vi "Read Stdout.vi"(8 "error in":errorcluster, 10 "byte count":i32, 11 "pipe in":T1) -> (0 "error out":errorcluster, 1 "return count":i32, 2 "read buffer":string, 3 "pipe out":T1, 4 "exited?":bool, 5 "bytes remaining":i32)   [LabVIEW 2013, in "LV Process library.lvlib"]
doc: "Calls lv_proc.dll to read stdout of a process and returns read buffer. Also returns count of remaining bytes in the pipe and process status. If process is not running, exited terminal is set to true.\n\n---\nLV Process works only with lv_proc.dll library, which is part of vipm package or should be delivered together with packed library. Placement of this dll is selected in terminal of Create Process.vi."
uses:
  LV Process library.lvlib
  Pipe Handle.ctl
panel:
  in  "exit mem":i32
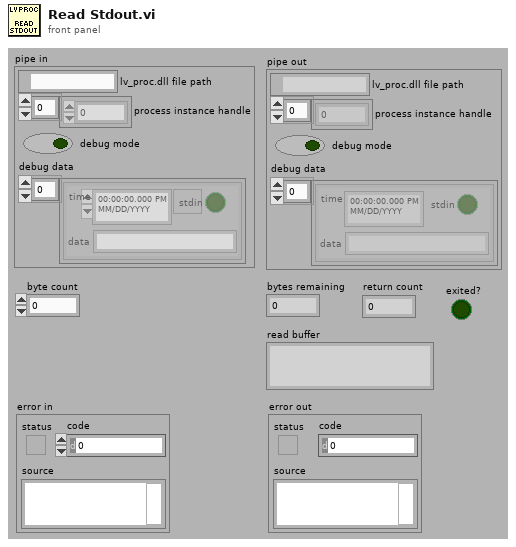
[diagram p1: front panel]
types:
  T1 = typedef "LV Process library.lvlib/Pipe Handle.ctl" = cluster{"lv_proc.dll file path":path, "process instance handle":u32[], "debug mode":bool, "debug data":cluster{"time":timestamp, "stdin":bool, "data":string}[]}
  T2 = cluster{"time":timestamp, "stdin":bool, "data":string}[]
  T3 = cluster{"time":timestamp, "stdin":bool, "data":string}
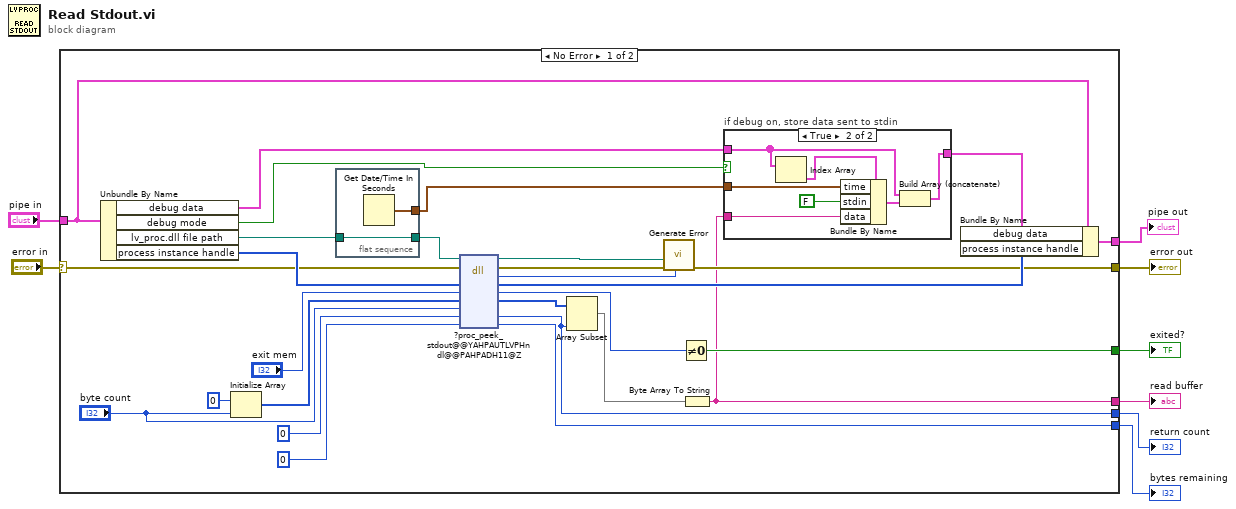
[diagram p0: block diagram]
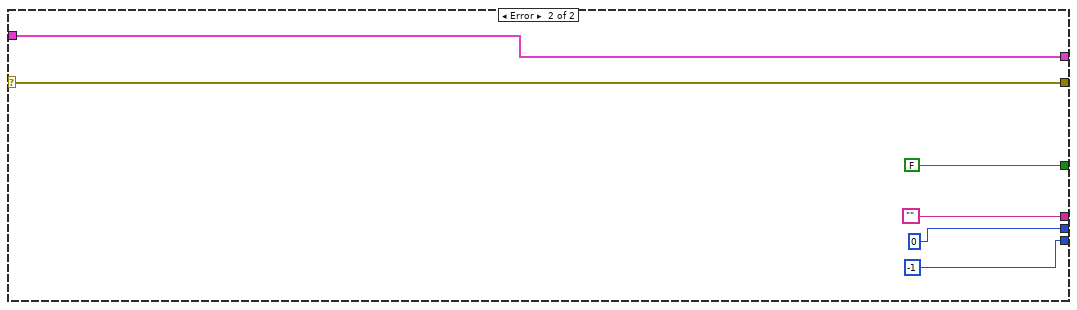
[diagram p3: hidden frame]
diagram:
  n1 = case shown="No Error" "error in" {
    selector: "error in" -> [w19 w52]
    tunnel: [w27 w51] -> w8
    tunnel: "pipe in" -> [w26 w51]
    tunnel: [w20 w52] -> w6
    tunnel: [w10 ""] -> w4
    tunnel: [w18 FALSE] -> w3
    tunnel: [w17 0 ("read")] -> w2
    tunnel: [w16 -1 ("toread")] -> w1
    frame No Error {
      n2 = Unbundle By Name(w26) -> ("debug data"=w14:T2, "debug mode"=w15:bool, "lv_proc.dll file path"=w13:path, "process instance handle"=w23:u32[])
      n3 = Initialize Array(u8 0 ("element"), "byte count") -> (w33:u8[])
      n4 = flat-sequence {
        tunnel: [w38] -> w12
        tunnel: w13 -> [w38]
        tunnel: [w37] -> w11
        frame #0 {
          n5 = Get Date/Time In Seconds() -> (seconds since 1Jan1904=w37:timestamp)
        }
      }
      n6 = dll-call lib="C:/Data/GOLPI/LV Process/lv_proc.dll" fn="?proc_peek_stdout@@YAHPAUTLVPHndl@@PAHPADH11@Z" label="proc_peek_stdout"(path in=w12, error in=w19, "proc"=w23, "exit"="exit mem", "buffer"=w33, "size"="byte count", "read"=0 ("read mem"), "toread"=0 ("toread mem")) -> (path out=w22:path, error out=w21:errorcluster, "error"=w24:i32, "proc"=w25:u32[], "exit"=w30:i32, "buffer"=w29:u8[], "read"=w17:i32, "toread"=w16:i32)  [unwired: 2 in]
      n7 = Array Subset(array=w29, length=w17) -> (w28:u8[])  [unwired: 1 in]
      n8 = call "Generate Error.vi"("error code in"=w24, "error in"=w21, "lv_proc.dll path in"=w22) -> ("error out"=w20:errorcluster)  [unwired: 6 in, 1 out]
      n9 = Not Equal To 0?(x=w30) -> (x != 0?=w18:bool)
      n10 = Byte Array To String(unsigned byte array=w28) -> (string=w10:string)
      n11 = case "if debug on, store data sent to stdin" shown="True" w15 {
        tunnel: w14 -> [w39 w45]
        tunnel: w11 -> [_ w42]
        tunnel: w10 -> [_ w41]
        tunnel: [w39 w40] -> w9
        frame False {
        }
        frame True {
          n12 = Index Array(array=w45) -> (element=w46:T3)  [unwired: 1 in]
          n13 = Bundle By Name(cluster=w46, "time"=w42, "stdin"=FALSE, "data"=w41) -> (w44:T3)
          n14 = Build Array (concatenate)(w45, w44) -> (w40:T2)
        }
      }
      n15 = Bundle By Name(cluster=w26, "debug data"=w9, "process instance handle"=w25) -> (w27:T1)
    }
    frame Error {
    }
  }
  "error out" <- w6
  "pipe out" <- w8
  "read buffer" <- w4
  "exited?" <- w3
  "return count" <- w2
  "bytes remaining" <- w1
